vi "FreshSingleItem.vi"(8 "error in (no error)":errorcluster, 10 "TableItem":refnum<vi>, 11 "TableItem in":refnum<class "TableItem.lvclass">) -> (0 "error out":errorcluster, 3 "TableItem out":refnum<class "TableItem.lvclass">)   [LabVIEW 2015, in "ActorManagement.lvlib" / "TableItem.lvclass"]
uses:
  TableItem.lvclass
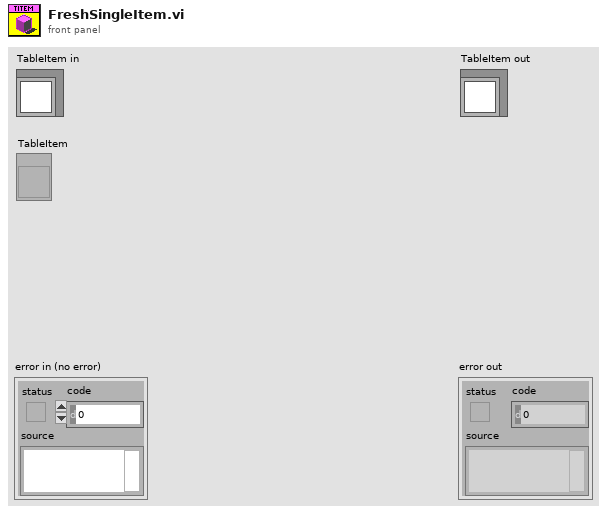
[diagram p1: front panel]
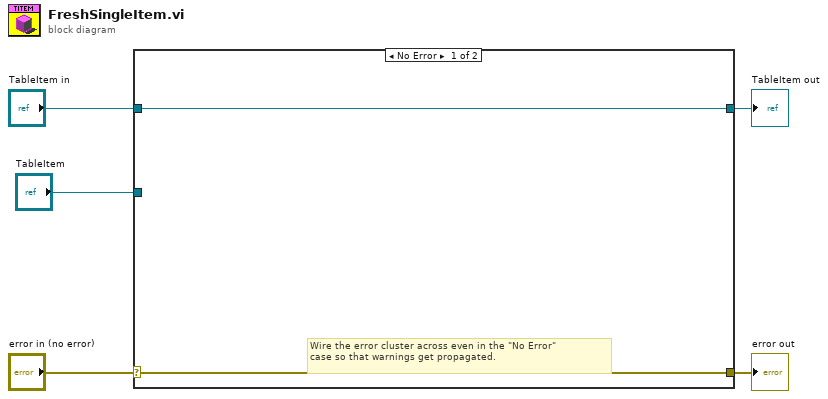
[diagram p0: block diagram]
diagram:
  n1 = case shown="No Error" "error in (no error)" {
    selector: "error in (no error)" -> [w6 w9]
    tunnel: [w6 w9] -> w4
    tunnel: [w7 w8] -> w2
    tunnel: "TableItem in" -> [w7 w8]
    tunnel: "TableItem" -> [_ _]
    frame No Error {
      # "Wire the error cluster across even in the \"No Error\"\ncase so that warnings get propagated."
    }
    frame Error {
    }
  }
  "error out" <- w4
  "TableItem out" <- w2
